vi "TransferItems.vi"(8 "error in (no error)":errorcluster, 10 "Session":refnum<class "Session.lvclass">, 11 "TransferFolder in":refnum<class "TransferFolder.lvclass">) -> (0 "error out":errorcluster, 3 "FileTransfer out":refnum<class "TransferFolder.lvclass">)   [LabVIEW 2015, in "WinSCP.lvlib" / "TransferFolder.lvclass"]
uses:
  TransferFolder.lvclass
  Session/Session.lvclass
  FileTransferOptions/FileTransferOptions.lvclass
  C:/Program Files (x86)/WinSCP/WinSCPnet.dll
  Program Files (x86)/WinSCP/WinSCPnet.dll
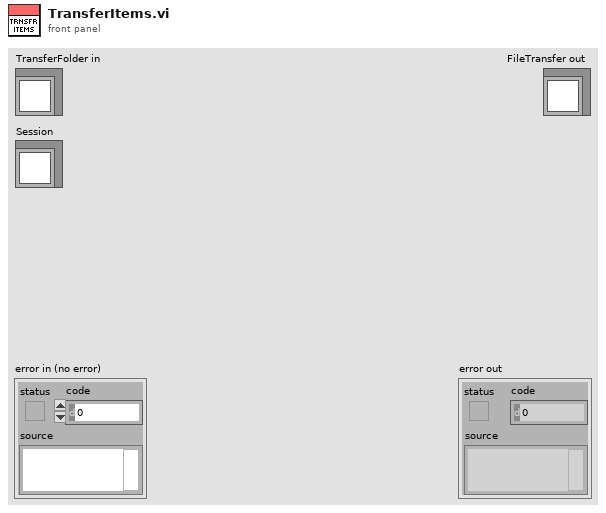
[diagram p1: front panel]
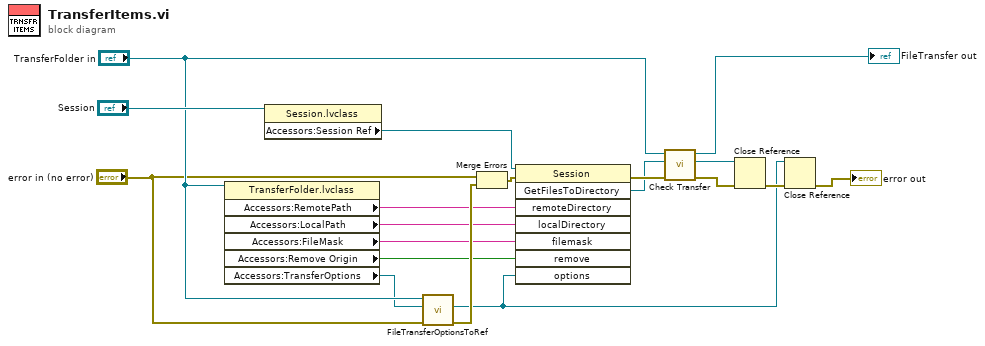
[diagram p0: block diagram]
diagram:
  n1 = property class="TransferFolder.lvclass"(reference="TransferFolder in") -> ("Accessors:RemotePath"=w18:string, "Accessors:LocalPath"=w17:string, "Accessors:FileMask"=w16:string, "Accessors:Remove Origin"=w15:bool, "Accessors:TransferOptions"=w6:refnum<class "FileTransferOptions.lvclass">)  [unwired: 1 in, 2 out]
  n2 = property class="Session.lvclass"(reference="Session") -> ("Accessors:Session Ref"=w11:refnum<k24>)  [unwired: 1 in, 2 out]
  n3 = call-dynamic "FileTransferOptionsToRef.vi"("error in (no error)"="error in (no error)", "FileTransferOptions"=w6, "FileTransfer in"="TransferFolder in") -> ("error out"=w19:errorcluster, "TransferOptions Ref"=w3:refnum<k24>)  [unwired: 7 in]
  n4 = Merge Errors("error in (no error)", w19) -> (w1:errorcluster)
  n5 = invoke class="Session" method="GetFilesToDirectory"(reference=w11, error in=w1, "remoteDirectory"=w18, "localDirectory"=w17, "filemask"=w16, "remove"=w15, "options"=w3) -> (error out=w14:errorcluster, "GetFilesToDirectory"=w13:refnum<k24>)  [unwired: 1 in, 6 out]
  n6 = call-dynamic "Check Transfer.vi"("error in"=w14, "TransferOperationResult in"=w13, "FileTransfer in"="TransferFolder in") -> ("error out"=w9:errorcluster, "TransferOperationResult out"=w10:refnum<k24>, "FileTransfer out"=→"FileTransfer out":refnum<class "TransferFolder.lvclass">)  [unwired: 6 in]
  n7 = Close Reference(reference=w10, error in (no error)=w9) -> (error out=w5:errorcluster)
  n8 = Close Reference(reference=w3, error in (no error)=w5) -> (error out=→"error out":errorcluster)
